vi "Install Server.vi"() -> ()   [LabVIEW 2025, in "Tools.lvlib"]
uses:
  Tools.lvlib
  <vilib>/Utility/sysdir.llb/System Directory Type.ctl
  <vilib>/Platform/browser.llb/Open URL in Default Browser (string).vi
panel:
  out "text":string
  out "system directory":path
  in  "Install MCP Server":bool
  in  "Install Python Packages":bool
  in  "Install Python":bool
  # "1.\n\n2.\n\n3."
  # "1. Install Python\n2. Install packages\n-mcp[cli]\n-pywin32\n3. Add server python-file to Claude Desktop"
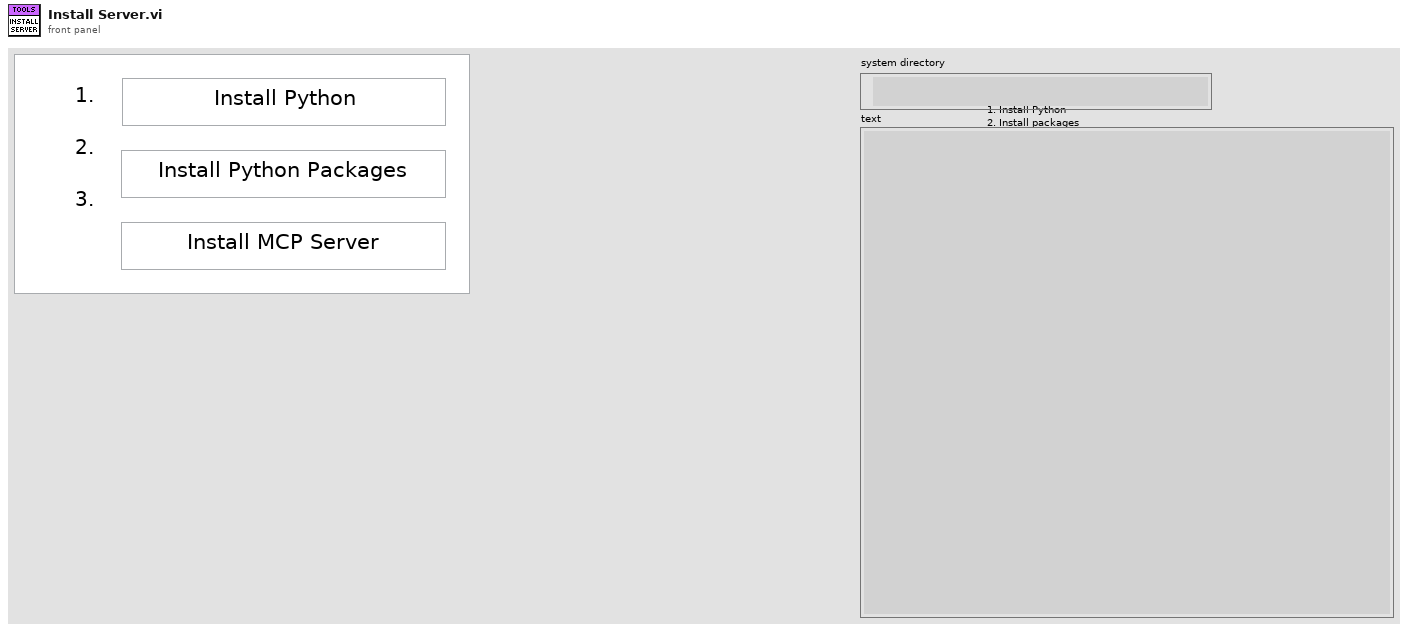
[diagram p1: front panel]
types:
  T1 = enum16{"open", "replace", "create", "open or create", "replace or create", "replace or create with confirmation"}
  T2 = typedef "System Directory Type.ctl" = i32
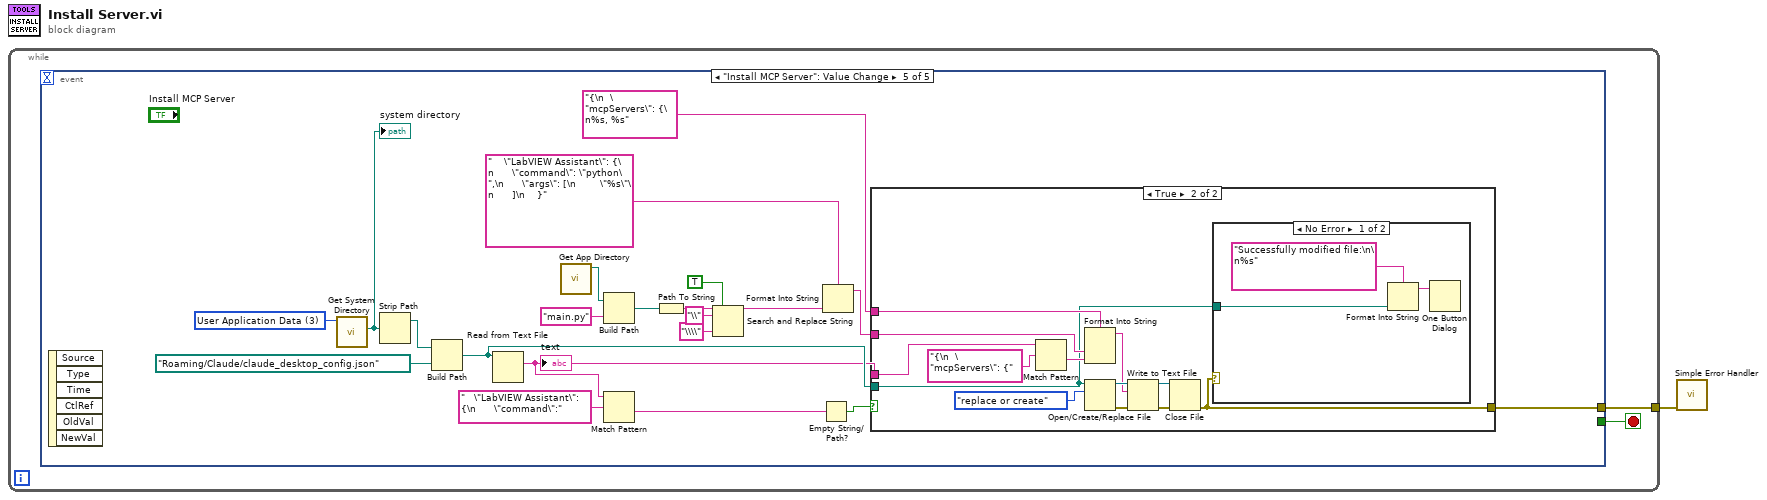
[diagram p0: block diagram]
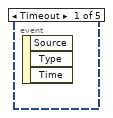
[diagram p2: hidden frame]
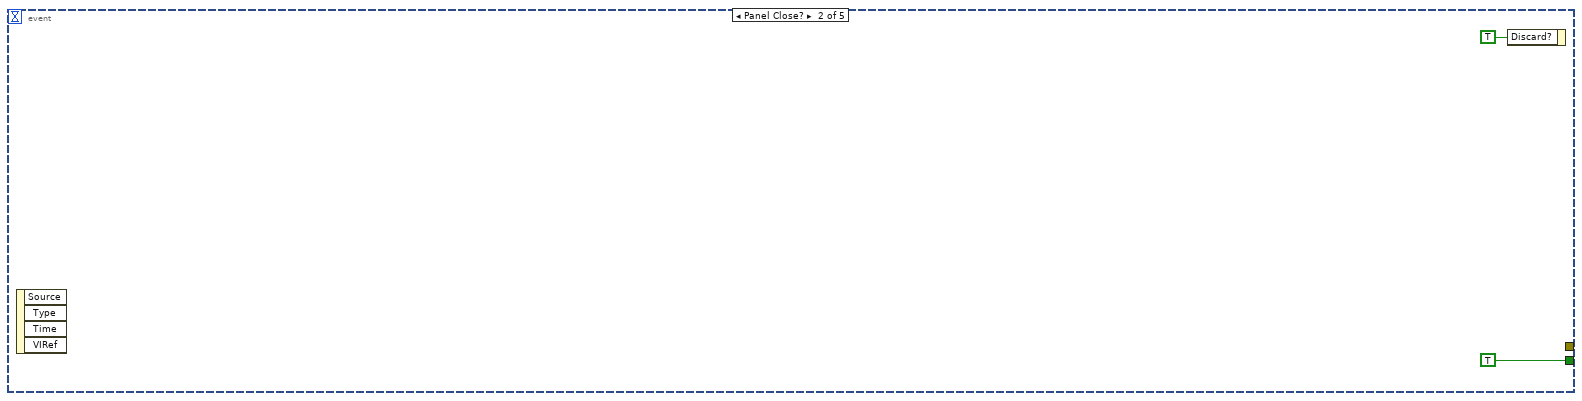
[diagram p3: hidden frame]
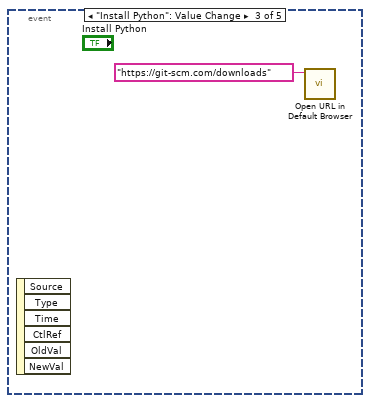
[diagram p4: hidden frame]
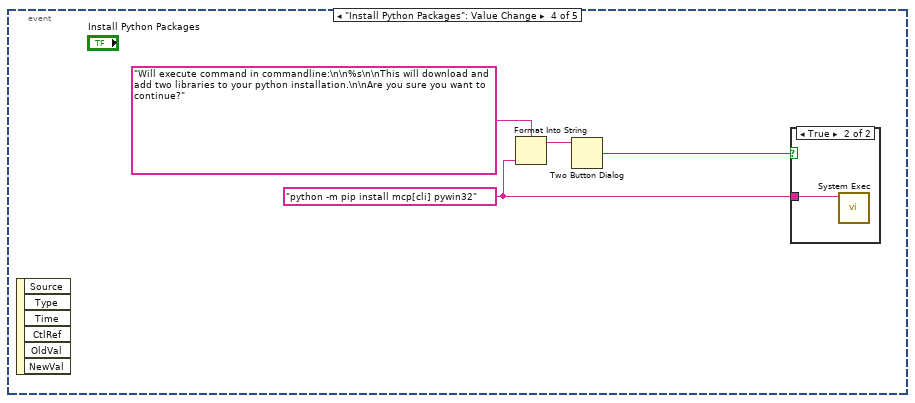
[diagram p5: hidden frame]
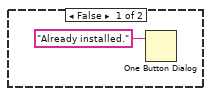
[diagram p7: hidden frame]
diagram:
  n1 = while {
    tunnel: [w2] -> w1
    stop <- w3 stop-if-true
    n2 = event shown="[4] \"Install MCP Server\": Value Change" {
      selector: _ -> [_ _ _ _ _]
      dyn-events: _ -> [_ _ _ _ _]
      timeout: _ -> [_ _ _ _ _]
      tunnel: [_ TRUE ("Discard?") _ _ _] -> w3
      tunnel: [_ _ _ _ w27] -> w2
      event Timeout {
        n3 = event-data() -> ()  [unwired: 1 in, 3 out]
      }
      event Panel Close? {
        n4 = event-data() -> ()  [unwired: 1 in, 4 out]
        n5 = event-data("Discard?"=TRUE) -> ()  [unwired: 1 in, 1 out]
      }
      event "Install Python": Value Change {
        n6 = event-data() -> ()  [unwired: 1 in, 6 out]
        n7 = call-poly <vilib>:"Open URL in Default Browser.vi"("URL"="https://git-scm.com/downloads") -> ()  [unwired: 5 in, 2 out]
      }
      event "Install Python Packages": Value Change {
        w8 = "python -m pip install mcp[cli] pywin32" ("input 1")
        n8 = event-data() -> ()  [unwired: 1 in, 6 out]
        n9 = Format Into String(format string="Will execute command in commandline:\n\n%s\n\nThis will download and add two libraries to your python installation.\n\nAre you sure you want to continue?" ("message"), w8) -> (resulting string=w9:string)  [unwired: 2 in, 1 out]
        n10 = Two Button Dialog(message=w9) -> (T button?=w7:bool)  [unwired: 2 in]
        n11 = case shown="True" w7 {
          tunnel: w8 -> [_ w11]
          frame False {
          }
          frame True {
            n12 = call <vilib>:"System Exec.vi"("command line"=w11) -> ()  [unwired: 7 in, 4 out]
          }
        }
      }
      event "Install MCP Server": Value Change {
        w32 = T2 3 items=["User Home"=0, "User Desktop"=1, "User Documents"=2, "User Application Data"=3, "User Preferences"=4, "User Temporary"=5, "Public Documents"=6, "Public Application Data"=7, "Public Preferences"=8, "Public Cache"=13, "System Core Libraries"=9, "System Installed Libraries"=10, "Application Files"=11, "Boot Volume Root"=12] ("system directory type")
        n13 = event-data() -> ()  [unwired: 1 in, 6 out]
        n14 = call <vilib>:"Get System Directory.vi"("system directory type"=w32) -> ("system directory"=w21:path)  [unwired: 10 in]
        "system directory" <- w21
        n15 = Strip Path(path=w21) -> (stripped path=w31:path)  [unwired: 1 out]
        n16 = Build Path(base path=w31, name or relative path=path "Roaming/Claude/claude_desktop_config.json") -> (appended path=w28:path)
        n17 = Read from Text File(file (use dialog)=w28) -> (text=w25:string)  [unwired: 3 in, 3 out]
        "text" <- w25
        n18 = call "Get App Directory.vi"() -> ("appended path"=w19:path)  [unwired: 11 in]
        n19 = Build Path(base path=w19, name or relative path="main.py" ("message")) -> (appended path=w20:path)
        n20 = Match Pattern(string=w25, regular expression="   \"LabVIEW Assistant\": {\n      \"command\":") -> (after substring=w24:string)  [unwired: 1 in, 3 out]
        n21 = Path To String(path=w20) -> (string=w16:string)
        n22 = Search and Replace String(replace all?=TRUE ("replace all? (F)"), input string=w16, search string="\\", replace string="\\\\" ("replace string (\"\")")) -> (result string=w13:string)  [unwired: 4 in, 3 out]
        n23 = Empty String/Path?(string/path=w24) -> (empty?=w23:bool)
        n24 = Format Into String(format string="    \"LabVIEW Assistant\": {\n      \"command\": \"python\",\n      \"args\": [\n        \"%s\"\n      ]\n    }" ("message"), w13) -> (resulting string=w17:string)  [unwired: 2 in, 1 out]
        n25 = case shown="True" w23 {
          tunnel: "{\n  \"mcpServers\": {\n%s, %s" ("regular expression") -> [_ w45]
          tunnel: w17 -> [_ w44]
          tunnel: w28 -> [_ w34]
          tunnel: [_ w35] -> w27
          tunnel: w25 -> [_ w41]
          frame False {
            n26 = One Button Dialog(message="Already installed.") -> ()  [unwired: 1 in, 1 out]
          }
          frame True {
            n27 = Match Pattern(string=w41, regular expression="{\n  \"mcpServers\": {") -> (after substring=w43:string)  [unwired: 1 in, 3 out]
            n28 = Format Into String(format string=w45, w44, w43) -> (resulting string=w36:string)  [unwired: 2 in, 1 out]
            n29 = Open/Create/Replace File(file path (use dialog)=w34, operation (0:open)=T1."replace or create") -> (refnum out=w40:refnum<file>, error out=w38:errorcluster)  [unwired: 4 in, 1 out]
            n30 = Write to Text File(file (use dialog)=w40, text=w36, error in=w38) -> (refnum out=w37:refnum<file>, error out=w39:errorcluster)  [unwired: 1 in, 1 out]
            n31 = Close File(refnum=w37, error in=w39) -> (error out=w35:errorcluster)  [unwired: 1 out]
            n32 = case shown="No Error" w35 {
              tunnel: w34 -> [w48 _]
              frame No Error {
                n33 = Format Into String(format string="Successfully modified file:\n\n%s" ("message"), w48) -> (resulting string=w47:string)  [unwired: 2 in, 1 out]
                n34 = One Button Dialog(message=w47) -> ()  [unwired: 1 in, 1 out]
              }
              frame Error {
              }
            }
          }
        }
      }
    }
  }
  n35 = call <vilib>:"Simple Error Handler.vi"("error in (no error)"=w1) -> ()  [unwired: 4 in, 5 out]
